vi "host.vi"() -> ()   [LabVIEW 2020]
uses:
  b4957acc-33c7-4f51-b6c8-be02e890b770.vi
  <vilib>/Array/Sort 2D Array - Pop Stack.vi
  <vilib>/Array/Sort 2D Array - Push Stack.vi
  b4957acc-33c7-4f51-b6c8-be02e890b770.vi/269d4b3b-47f5-49e3-8884-44851e4dd9d5.vi
  b4957acc-33c7-4f51-b6c8-be02e890b770.vi/6d99389c-673d-4efb-bf33-19b32bcf4cf8.vi
  <vilib>/FPGAPlugInAG/cRIO-9035/niLvFpga_Open_cRIO-9035.vi
  <vilib>/FPGAPlugInAG/cRIO-9035/niLvFpga_Reset_cRIO-9035.vi
  <vilib>/Utility/error.llb/Error Cluster From Error Code.vi
  <vilib>/rvi/errors/niLvFpgaAdjustHostInterfaceError.vi
  <vilib>/FPGAPlugInAG/cRIO-9035/niLvFpga_Run_cRIO-9035.vi
  <vilib>/FPGAPlugInAG/cRIO-9035/niLvFpga_Close_cRIO-9035.vi
  <vilib>/rvi/interface/nirviOpenFPGA/nirviOpenFPGA.xnode
  FPGA Bitfiles/project_FPGATarget_target_Og4RcSvXPjM.lvbitx
  target.vi
  <vilib>/rvi/interface/nirviMethod/nirviMethod.xnode
  <vilib>/rvi/interface/nirviReadWriteControl/nirviReadWriteControl.xnode
  <vilib>/rvi/interface/nirviCloseFPGA/nirviCloseFPGA.xnode
  <vilib>/Analysis/NI_AALBase.lvlib
  <vilib>/FPGAPlugInAG/cRIO-9035/niLvFpga_StartFifo_cRIO-9035.vi
  <vilib>/rvi/errors/niLvFpgaMergeErrorWithErrorCode.vi
  <vilib>/FPGAPlugInAG/cRIO-9035/niLvFpga_ReadFifo_cRIO-9035.vi
  <vilib>/FPGAPlugInAG/cRIO-9035/niLvFpga_WriteFifo_cRIO-9035.vi
  NiFpgaLv.dll
panel:
  out "Data":sgl[](array[numeric])
  out "error out":errorcluster
  out "Timed Out? FIFO out IMG":bool
  out "Timed Out? FIFO out REAL":bool
  out "Timed Out? FIFO in REAL":bool
  out "index values":i32[](array[numeric])
  out "sorted 2D array":sgl[][](array[numeric])
  out "input data":sgl[](graph)
  out "sort time (ms)":dbl
  out "Elements Remaining":u32
  out "Real sorted signal":sgl[](graph)
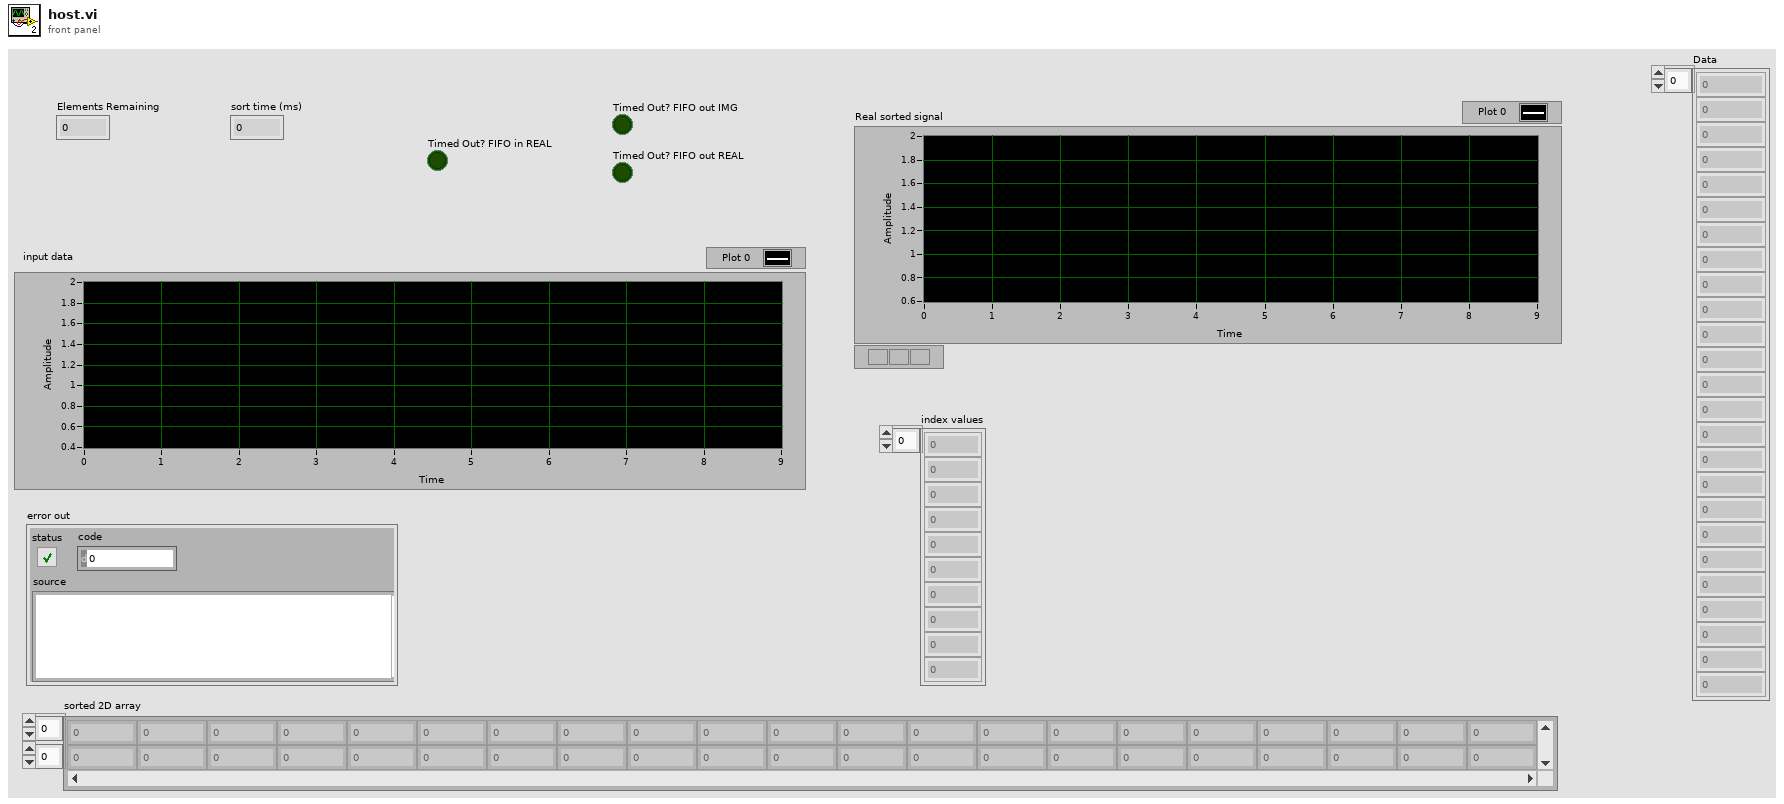
[diagram p1: front panel]
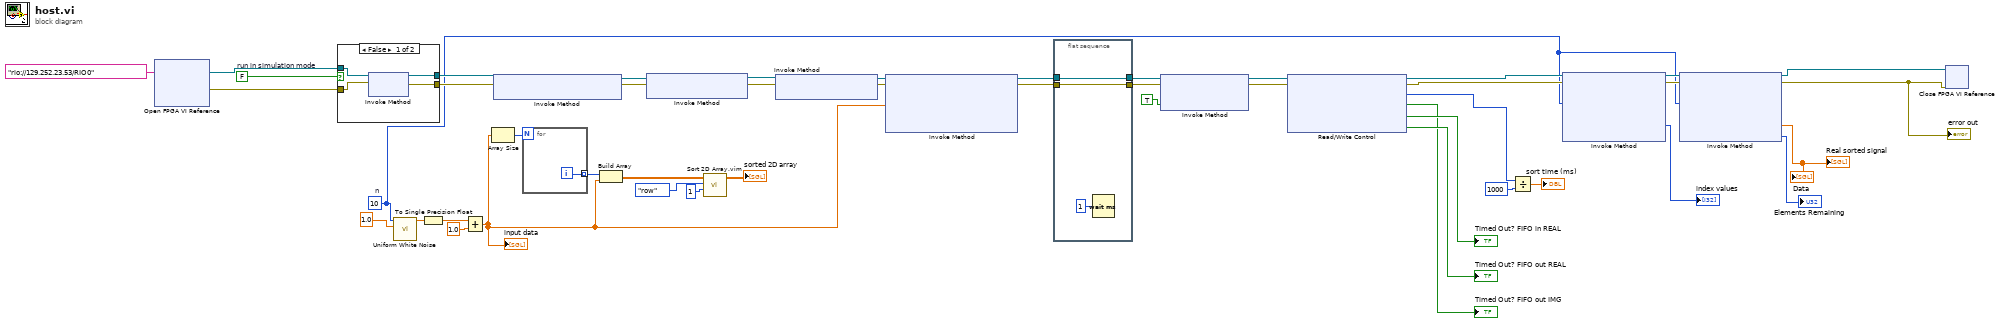
[diagram p0: block diagram]
diagram:
  w11 = FALSE  # run in simulation mode
  w1 = 10  # n
  n1 = xnode "Open FPGA VI Reference"("resource name"=tag "rio://129.252.23.53/RIO0") -> ("FPGA VI Reference Out"=w10:refnum<k20>, "error out"=w9:errorcluster)  [unwired: 1 in]
  n2 = case shown="False" w11 {
    tunnel: w10 -> [w50 w51]
    tunnel: w9 -> [w49 w52]
    tunnel: [w48 w51] -> w8
    tunnel: [w47 w52] -> w7
    frame False {
      n3 = xnode "Invoke Method"("FPGA VI Reference In"=w50, "error in"=w49) -> ("FPGA VI Reference Out"=w48:refnum<k20>, "error out"=w47:errorcluster)
    }
    frame True {
    }
  }
  n4 = call <vilib>:"Uniform White Noise.vi"("amplitude"=1.0, "samples"=w1) -> ("uniform white noise"=w25:dbl[])  [unwired: 8 in, 1 out]
  n5 = To Single Precision Float(number=w25) -> (single precision float=w24:sgl[])
  n6 = Add(x=w24, y=sgl 1.0 ("amplitude")) -> (x+y=w6:sgl[])
  "input data" <- w6
  n7 = Array Size(array=w6) -> (size(s)=w30:i32)
  n8 = xnode "Invoke Method"("FPGA VI Reference In"=w8, "error in"=w7) -> ("FPGA VI Reference Out"=w23:refnum<k20>, "error out"=w22:errorcluster)
  n9 = for {
    N: w30 -> [_]
    tunnel: [w53] -> w29 mode=indexing
    i -> [w53]
  }
  n10 = Build Array(w29, w6) -> (w28:sgl[][])
  n11 = xnode "Invoke Method"("FPGA VI Reference In"=w23, "error in"=w22) -> ("FPGA VI Reference Out"=w16:refnum<k20>, "error out"=w17:errorcluster)
  n12 = call "Sort 2D Array.vim"("index"=1, "dimension to index (column)"=enum16{"column", "row"}."row", "2D array"=w28) -> ("sorted 2D array"=→"sorted 2D array":sgl[][])  [unwired: 7 in, 1 out]
  n13 = xnode "Invoke Method"("FPGA VI Reference In"=w16, "error in"=w17) -> ("FPGA VI Reference Out"=w21:refnum<k20>, "error out"=w20:errorcluster)
  n14 = xnode "Invoke Method"("FPGA VI Reference In"=w21, "error in"=w20, "Data"=w6) -> ("FPGA VI Reference Out"=w19:refnum<k20>, "error out"=w18:errorcluster)  [unwired: 1 in, 1 out]
  n15 = flat-sequence {
    tunnel: [w55] -> w13
    tunnel: w19 -> [w55]
    tunnel: [w54] -> w12
    tunnel: w18 -> [w54]
    frame #0 {
      n16 = Wait (ms)(milliseconds to wait=u32 1) -> ()  [unwired: 1 out]
    }
  }
  n17 = xnode "Invoke Method"("FPGA VI Reference In"=w13, "error in"=w12, "Wait Until Done (F)"=TRUE) -> ("FPGA VI Reference Out"=w43:refnum<k20>, "error out"=w42:errorcluster)
  n18 = xnode "Read/Write Control"("FPGA VI Reference In"=w43, "error in"=w42) -> ("FPGA VI Reference Out"=w37:refnum<k20>, "error out"=w35:errorcluster, "sort time (us)"=w41:u32, "Timed Out? FIFO out index"=→"Timed Out? FIFO out IMG":bool, "Timed Out? FIFO in REAL"=→"Timed Out? FIFO in REAL":bool, "Timed Out? FIFO out REAL"=→"Timed Out? FIFO out REAL":bool)
  n19 = Divide(x=w41, y=u32 1000) -> (x/y=→"sort time (ms)":dbl)
  n20 = xnode "Invoke Method"("FPGA VI Reference In"=w37, "error in"=w35, "Number of Elements"=w1) -> ("FPGA VI Reference Out"=w36:refnum<k20>, "error out"=w34:errorcluster, "Data"=→"index values":i32[])  [unwired: 1 in, 1 out]
  n21 = xnode "Invoke Method"("FPGA VI Reference In"=w36, "error in"=w34, "Number of Elements"=w1) -> ("FPGA VI Reference Out"=w4:refnum<k20>, "error out"=w3:errorcluster, "Data"=→"Real sorted signal" →"Data":sgl[], "Elements Remaining"=→"Elements Remaining":u32)  [unwired: 1 in]
  "error out" <- w3
  n22 = xnode "Close FPGA VI Reference"("FPGA VI Reference In"=w4, "error in"=w3) -> ()  [unwired: 1 out]
